vi "SetChartDataInput.vi"() -> (0 "ChartDataInput":enum16{"EUData", "RawData"}(ring))   [LabVIEW 2019]
uses:
  <vilib>/Utility/config.llb/Read Key (String).vi
  <vilib>/Utility/config.llb/NI_LVConfig.lvlib
panel:
  in  "Error In":errorcluster
  out "Error Out":errorcluster
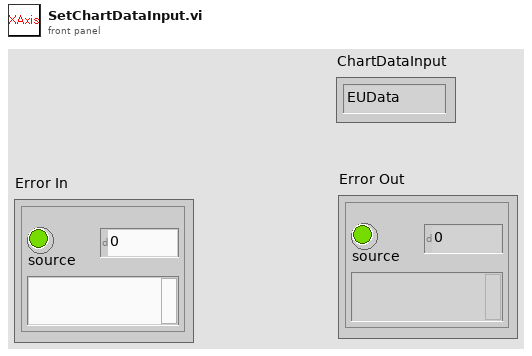
[diagram p1: front panel]
types:
  T1 = typedef "NI_LVConfig.lvlib/Config Data RefNum.ctl" = refnum<k1>
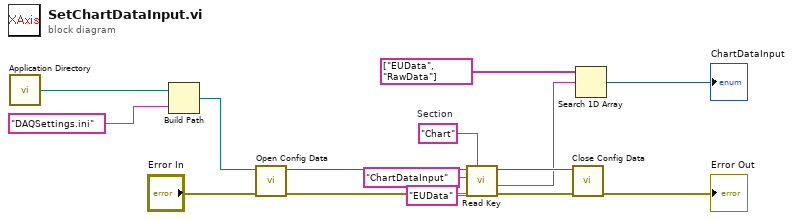
[diagram p0: block diagram]
diagram:
  w11 = "Chart"  # Section
  n1 = call <vilib>:"Application Directory.vi"() -> ("Application Directory"=w15:path)
  n2 = Build Path(base path=w15, name or relative path="DAQSettings.ini") -> (appended path=w13:path)
  n3 = call <vilib>:"Open Config Data.vi"("error in (no error)"="Error In", "configuration file path"=w13) -> ("error out"=w3:errorcluster, "refnum"=w8:T1)  [unwired: 7 in, 1 out]
  n4 = call-poly <vilib>:"Read Key.vi"("section"=w11, "error in (no error)"=w3, "default value"="EUData", "key"="ChartDataInput", "refnum"=w8) -> ("error out"=w9:errorcluster, "value"=w4:string, "refnum out"=w10:T1)  [unwired: 3 in, 1 out]
  n5 = call <vilib>:"Close Config Data.vi"("error in (no error)"=w9, "refnum"=w10) -> ("error out"=→"Error Out":errorcluster)  [unwired: 8 in, 1 out]
  n6 = Search 1D Array(1D array=string[] ["EUData", "RawData"], element=w4) -> (index of element=→"ChartDataInput":i32)  [unwired: 1 in]
